vi "Extract value using keyword.vi"(0 "Keyword":string, 3 "Header":string[](array[string])) -> (14 "Value":string)   [LabVIEW 2022 SP3, in "RPC.lvclass"]
uses:
  RPC.lvclass
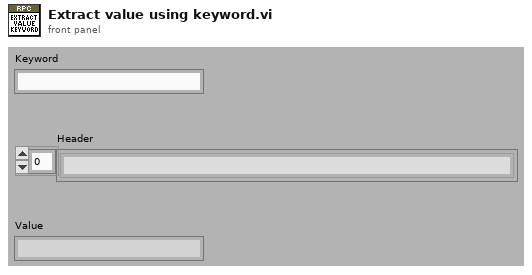
[diagram p1: front panel]
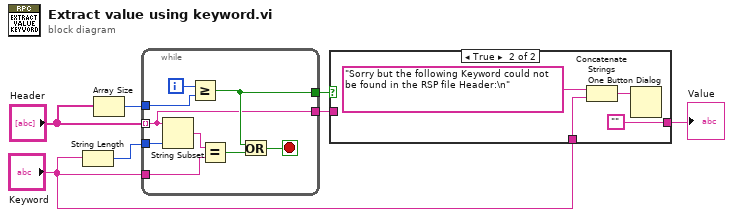
[diagram p0: block diagram]
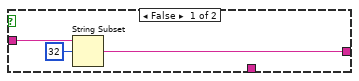
[diagram p2: hidden frame]
diagram:
  n1 = String Length(string="Keyword") -> (length=w7:i32)
  n2 = Array Size(array="Header") -> (size(s)=w5:i32)
  n3 = while {
    tunnel: "Header" -> [w8] mode=indexing
    tunnel: w7 -> [w16]
    tunnel: "Keyword" -> [w15]
    tunnel: w5 -> [w10]
    tunnel: [w9] -> w4
    tunnel: [w8] -> w2
    i -> [w11]
    stop <- w12 stop-if-true
    n4 = String Subset(string=w8, length (rest)=w16) -> (substring=w14:string)  [unwired: 1 out]
    n5 = Greater Or Equal?(x=w11, y=w10) -> (x >= y?=w9:bool)
    n6 = Equal?(x=w14, y=w15) -> (x = y?=w13:bool)
    n7 = Or(x=w9, y=w13) -> (x .or. y?=w12:bool)
  }
  n8 = case shown="True" w4 {
    tunnel: "Keyword" -> [_ w23]
    tunnel: w2 -> [w19 _]
    tunnel: [w17 ""] -> w1
    frame False {
      n9 = String Subset(string=w19, offset (0)=32) -> (substring=w17:string)  [unwired: 1 out]
    }
    frame True {
      n10 = Concatenate Strings("Sorry but the following Keyword could not be found in the RSP file Header:\n", w23) -> (w22:string)
      n11 = One Button Dialog(message=w22) -> ()  [unwired: 2 out]
    }
  }
  "Value" <- w1
